vi "Initialize.vi"(6 "optional":variant, 8 "error in":errorcluster, 11 "xceNode in":refnum<class "xceNode.lvclass">) -> (0 "error out":errorcluster, 3 "Node*":refnum<data-value>)   [LabVIEW 2013, in "xceNode.lvclass"]
doc: "Initializes a node. Makes a data value reference of the node, sets the selfNode, and output the data value reference."
uses:
  xceNode.lvclass
  xceNode.lvclass/xceNode.ctl
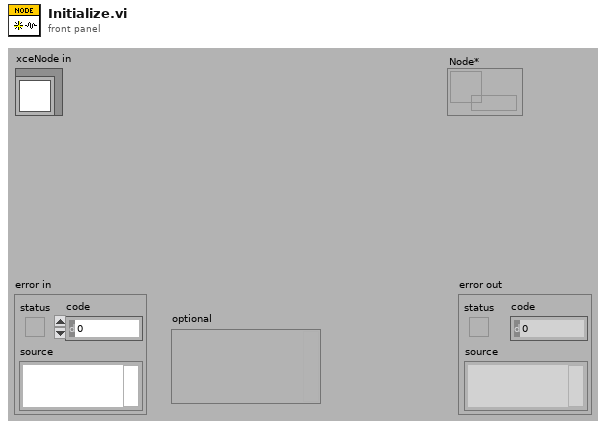
[diagram p1: front panel]
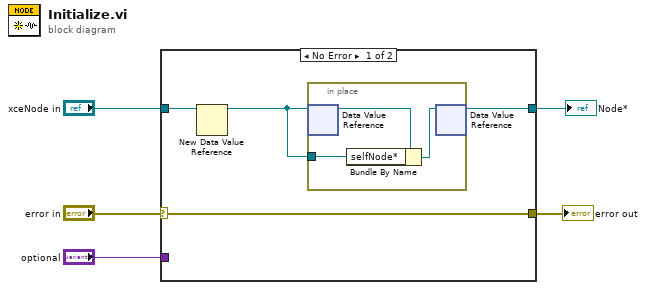
[diagram p0: block diagram]
diagram:
  n1 = case shown="No Error" "error in" {
    selector: "error in" -> [w9 w13]
    tunnel: [w9 w13] -> w4
    tunnel: "xceNode in" -> [w8 _]
    tunnel: "optional" -> [_ _]
    tunnel: [w7 _] -> w1
    frame No Error {
      n2 = New Data Value Reference(data value=w8) -> (data value reference=w6:refnum<data-value>)  [unwired: 1 in, 1 out]
      n3 = in-place {
        in-place-border: w6 -> [w11]
        n4 = in-place-dvr #1(w6) -> (w12:refnum<class "xceNode.lvclass">)  [unwired: 1 out]
        n5 = Bundle By Name(cluster=w12, "selfNode*"=w11) -> (w10:refnum<class "xceNode.lvclass">)
        n6 = in-place-dvr #1(w10) -> (w7:refnum<data-value>)  [unwired: 1 out]
      }
    }
    frame Error {
    }
  }
  "error out" <- w4
  "Node*" <- w1
